vi "Measuring Complete - AndreTec-4.vi"() -> ()   [LabVIEW 2014]
doc: "André Romero - 2016\nandretec@ifsc.usp.br\nIFSC - USP"
uses:
  <vilib>/Analysis/Matrix/Datatypes/RealMatrix.ctl
  C:/UserLabs/Andre/Nova-Autolab/Labview/Autolab SDK 1.11/EcoChemie.Autolab.Sdk.dll
  EcoChemie.Autolab.Sdk.dll
  <vilib>/Instr/_visa.llb/VISA Configure Serial Port (Instr).vi
  <vilib>/Utility/file.llb/Write To Spreadsheet File (DBL).vi
  <vilib>/Analysis/Matrix/NI_Matrix.lvlib
panel:
  in  "String":string="Wait !!!! Instrument is initializing ...."
  in  "Start Measurement":bool
  out "Sensor":i32=1
  out "error out":errorcluster={"status"=TRUE, "code"=-1073807343, "source"="Property Node (arg 1) in VISA Configure Serial Port (Instr).vi->Measuring Complete - AndreTec-2.vi"}
  out "VISA resource name out":refnum<visa-resource-name>="COM3"
  in  "N. Sensors":i32=3 min=1 max=8
  out "Measurement":cluster{dbl[], dbl[]}(graph)
  out "Points":i32=478
  in  "Abort":bool
  in  "Y axis Signal":string(combo)="WE(1).Current"
  in  "X axis Signal":string(combo)="WE(1).Potential"
  out "Measured data":cluster{"Y":dbl[], "Y":dbl[]}[](graph)
  out "X axis value":dbl=-1.1810302734375e-08
  out "Y axis value":dbl=3.0517578124972244e-06
  out "Measurement active":bool
  out "Blacklisted Commands detected":bool
  in  "Load Procedure (.nox)":path=path "C:/Users/user/Documents/My Procedures 1.11/Procedures/bla.nox"
  out "Autolab Connected":bool
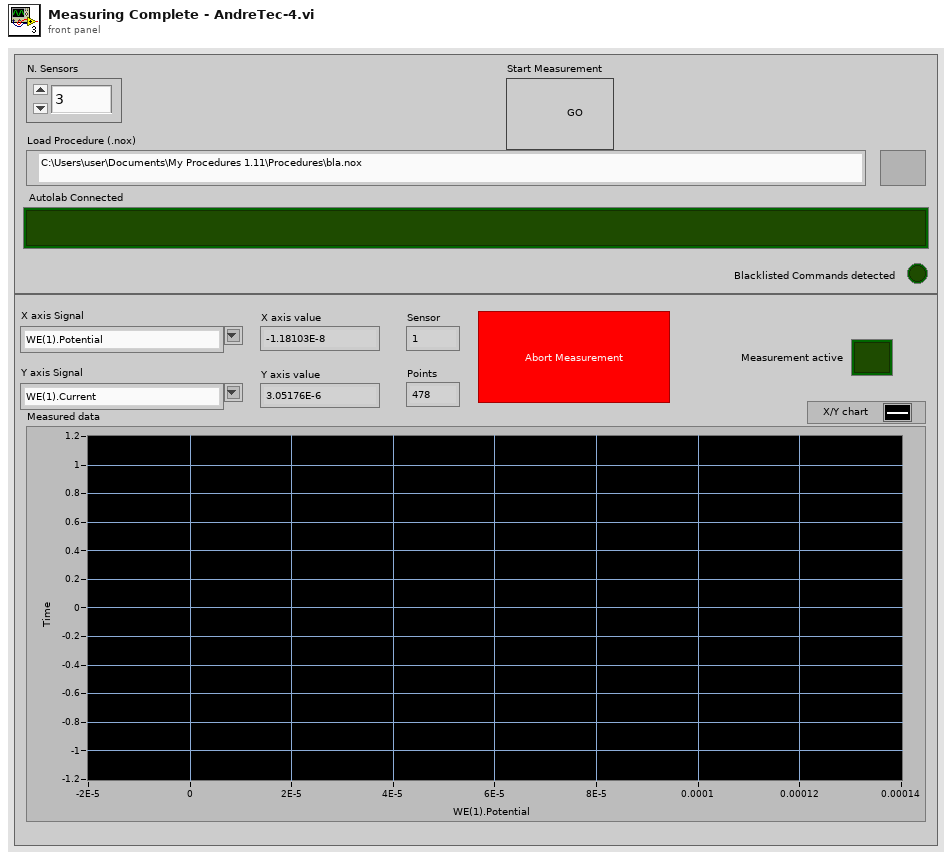
[diagram p1: front panel]
types:
  T1 = typedef "NI_Matrix.lvlib/RealMatrix.ctl" = dbl[][]
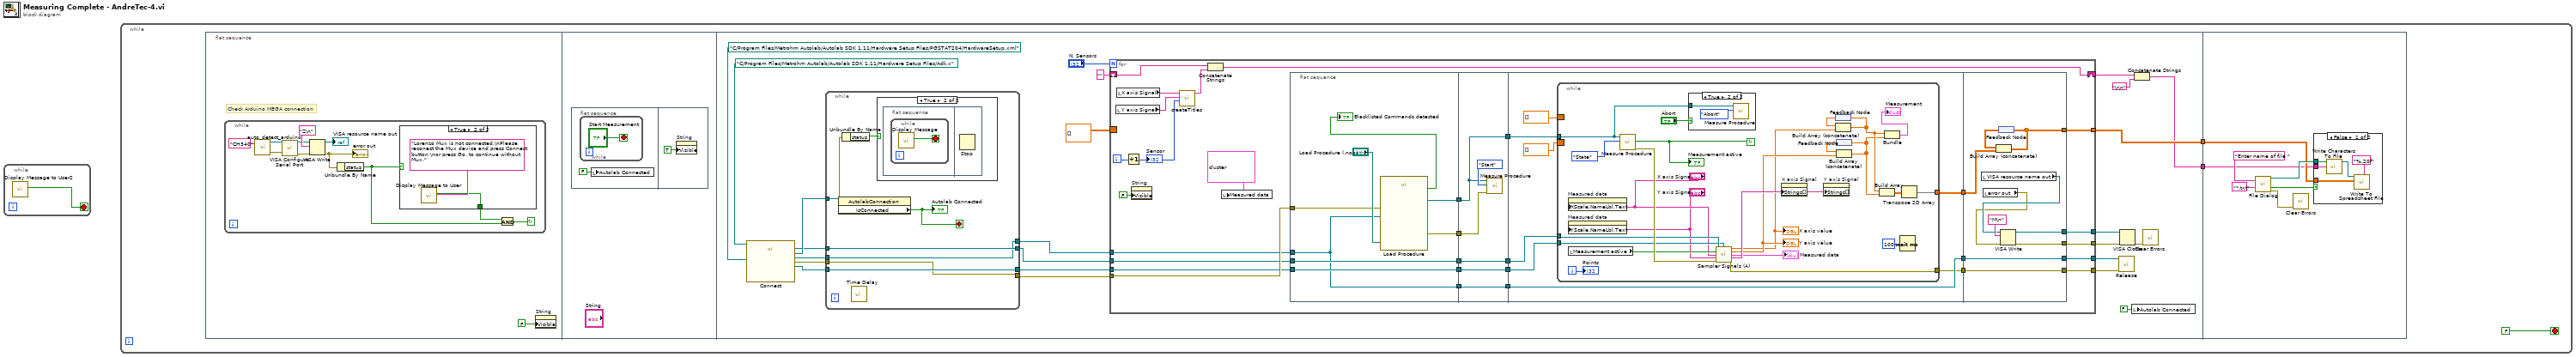
[diagram p0: block diagram]
diagram:
  n1 = while {
    stop <- w1 stop-if-true
    n2 = call "Display Message to User2"() -> ("OK"=w1:bool)  [unwired: 10 in, 1 out]
  }
  n3 = while {
    stop <- FALSE stop-if-true
    n4 = flat-sequence {
      tunnel: [w25] -> w3
      tunnel: [w23] -> w2
      tunnel: w3 -> [w146]
      tunnel: w2 -> [w145]
      frame #0 {
        # "Check Arduino MEGA connection"
        n5 = while {
          stop <- w8 continue-if-true
          n6 = call "auto_detect_arduino.vi"("instr name"="CH340") -> ("VISA resource name"=w16:refnum<visa-resource-name>, "error out"=w9:errorcluster)  [unwired: 1 in, 1 out]
          n7 = call-poly "VISA Configure Serial Port"("VISA resource name"=w16, "error in (no error)"=w9) -> ("VISA resource name out"=w13:refnum<visa-resource-name>, "error out"=w12:errorcluster)  [unwired: 7 in, 5 out]
          n8 = VISA Write(VISA resource name=w13, write buffer="Z\n" ("Command"), error in (no error)=w12) -> (VISA resource name out=→"VISA resource name out":refnum<visa-resource-name>, error out=w10:errorcluster)  [unwired: 1 out]
          "error out" <- w10
          n9 = Unbundle By Name(w10) -> ("status"=w7:bool)
          n10 = case shown="True" w7 {
            tunnel: [_ w17] -> w6
            frame False {
            }
            frame True {
              n11 = call "Display Message to User"("Message"="Lorenzo Mux is not connected.\nPlease reconect the Mux device and press Connect button \nor press Go, to continue without Mux.") -> ("Connect"=w17:bool)  [unwired: 9 in, 1 out]
            }
          }
          n12 = And(x=w6, y=w7) -> (x .and. y?=w8:bool)
        }
        n13 = property on="String" class="Str"("Visible"=FALSE) -> ()  [unwired: 2 in, 2 out]
      }
      frame #1 {
        n14 = flat-sequence {
          frame #0 {
            n15 = while {
              stop <- "Start Measurement" stop-if-true
            }
            n16 = local write "Autolab Connected"(FALSE ("Autolab Connected")) -> ()
          }
          frame #1 {
            n17 = property on="String" class="Str"("Visible"=TRUE) -> ()  [unwired: 2 in, 2 out]
          }
        }
      }
      frame #2 {
        n18 = call "Connect.vi"("Embedded Exe File"=path "C:/Program Files/Metrohm Autolab/Autolab SDK 1.11/Hardware Setup Files/Adk.x", "Hardware Setup File"=path "C:/Program Files/Metrohm Autolab/Autolab SDK 1.11/Hardware Setup Files/PGSTAT204/HardwareSetup.xml") -> ("Sampler"=w42:refnum<k24>, "AutolabConnection"=w43:refnum<k24>, "instrument"=w40:refnum<k24>, "Ei"=w35:refnum<k24>, "error out"=w37:errorcluster)  [unwired: 1 in, 8 out]
        n19 = while {
          tunnel: w43 -> [w140]
          tunnel: w42 -> [w137]
          tunnel: [w137] -> w41
          tunnel: w40 -> [w136]
          tunnel: [w136] -> w39
          tunnel: w35 -> [w135]
          tunnel: [w135] -> w38
          tunnel: w37 -> [w134]
          tunnel: [w134] -> w36
          stop <- w141 stop-if-true
          n20 = property class="AutolabConnection"(reference=w140) -> (error out=w138:errorcluster, "IsConnected"=w141:bool)  [unwired: 1 in, 1 out]
          "Autolab Connected" <- w141
          n21 = Unbundle By Name(w138) -> ("status"=w139:bool)
          n22 = call "Time Delay"() -> ()  [unwired: 2 in, 10 out]
          n23 = case shown="True" w139 {
            frame False {
            }
            frame True {
              n24 = flat-sequence {
                frame #0 {
                  n25 = while {
                    stop <- w142 stop-if-true
                    n26 = call "Display Message"() -> ("OK"=w142:bool)  [unwired: 10 in, 1 out]
                  }
                }
                frame #1 {
                  n27 = Stop() -> ()  [unwired: 1 in]
                }
              }
            }
          }
        }
        n28 = for {
          N: "N. Sensors" -> [_]
          tunnel: [w64] -> w34
          tunnel: [w63] -> w33
          tunnel: [w62] -> w30
          tunnel: [w61] -> w29
          tunnel: w36 -> [w60]
          tunnel: w39 -> [w59]
          tunnel: w41 -> [w58]
          tunnel: w38 -> [w57]
          tunnel: [w54] -> w25
          border: T1 [] ("Real Matrix") -> [_]
          shift-right: [w47] -> w24
          shift-left: "" -> [w49]
          i -> [w53]
          n29 = local read "Y axis Signal"() -> (w50:string)
          n30 = local read "X axis Signal"() -> (w51:string)
          n31 = Increment(x=w53) -> (x+1=w46:i32)
          "Sensor" <- w46
          n32 = property on="String" class="Str"("Visible"=FALSE) -> ()  [unwired: 2 in, 2 out]
          n33 = call "createTitles.vi"("Numeric"=w46, "Y axis Signal"=w50, "X axis Signal"=w51) -> ("String"=w48:string)  [unwired: 8 in]
          n34 = Concatenate Strings(w49, w48) -> (w47:string)
          n35 = local write "Measured data"(cluster{"Y":dbl[], "Y":dbl[]}[] [{"Y"=array[2393 elements], "Y"=array[2393 elements]}] ("Measured data")) -> ()
          n36 = flat-sequence {
            tunnel: [w81] -> w75
            tunnel: [w80] -> w74
            tunnel: [w78] -> w73
            tunnel: [w77] -> w72
            tunnel: [w76] -> w71
            tunnel: w59 -> [w76]
            tunnel: w60 -> [w79]
            tunnel: w58 -> [w78]
            tunnel: w57 -> [w77]
            tunnel: w75 -> [w87]
            tunnel: w74 -> [w88]
            tunnel: [w87] -> w70
            tunnel: w73 -> [w86]
            tunnel: w72 -> [w85]
            tunnel: [w86] -> w69
            tunnel: [w85] -> w68
            tunnel: [w84] -> w67
            tunnel: w71 -> [w84]
            tunnel: w70 -> [w97]
            tunnel: w69 -> [w96]
            tunnel: w68 -> [w95]
            tunnel: w67 -> [w94]
            tunnel: [w94] -> w66
            tunnel: [w90] -> w65
            tunnel: [w93] -> w55
            tunnel: w66 -> [w133]
            tunnel: w65 -> [w132]
            tunnel: [w133] -> w64
            tunnel: [w132] -> w63
            tunnel: [w128] -> w62
            tunnel: [w127] -> w61
            tunnel: w55 -> [w126]
            tunnel: [w124] -> w54
            frame #0 {
              n37 = call "Load Procedure.vi"("error in (no error)"=w79, "Procedure"="Load Procedure (.nox)", "Instrument"=w76) -> ("error out"=w80:errorcluster, "Contains"=→"Blacklisted Commands detected":bool, "LoadProcedure"=w81:refnum<k24>)  [unwired: 6 out]
            }
            frame #1 {
              n38 = call "Measure Procedure.vi"("error in"=w88, "Request for procedure"=enum16{"State", "Save", "Abort", "Start"}."Start", "LoadProcedure"=w87) -> ()  [unwired: 1 in, 8 out]
            }
            frame #2 {
              n39 = while {
                tunnel: w97 -> [w115]
                tunnel: w96 -> [w116]
                tunnel: w95 -> [w100]
                tunnel: [w103] -> w93
                border: dbl[] [] -> [_]
                border: dbl[] [] -> [_]
                tunnel: [w102] -> w90
                i -> [w112]
                stop <- w107 continue-if-true
                n40 = property on="Measured data" class="XYGraph (strict)"("XScale.NameLbl.Text"="X axis Signal") -> ()  [unwired: 2 in, 2 out]
                n41 = property on="Measured data" class="XYGraph (strict)"("YScale.NameLbl.Text"="Y axis Signal") -> ()  [unwired: 2 in, 2 out]
                n42 = local read "Measurement active"() -> (w118:bool)
                n43 = call "Measure Procedure.vi"("Request for procedure"=enum16{"State", "Save", "Abort", "Start"}."State", "LoadProcedure"=w115) -> ("error out"=w119:errorcluster, "IsMeasuring"=w107:bool)  [unwired: 2 in, 6 out]
                "Measurement active" <- w107
                n44 = case shown="True" "Abort" {
                  tunnel: w115 -> [_ w122]
                  frame False {
                  }
                  frame True {
                    n45 = call "Measure Procedure.vi"("Request for procedure"=enum16{"State", "Save", "Abort", "Start"}."Abort", "LoadProcedure"=w122) -> ()  [unwired: 2 in, 8 out]
                  }
                }
                n46 = call "Sampler Signals (A).vi"("IsMeasuring"=w118, "EI"=w100, "Sampler"=w116, "Signal X"="X axis Signal", "Signal Y"="Y axis Signal", "error in"=w119) -> ("X"=w101:dbl, "Y"=w109:dbl, "XY Graph"=→"Measured data":cluster{"Y":dbl[], "Y":dbl[]}[], "GetSignals"=w121:string[], "error out"=w102:errorcluster)  [unwired: 4 in, 1 out]
                "Y axis value" <- w109
                "X axis value" <- w101
                n47 = property on="X axis Signal" class="CmbBox"("Strings[]"=w121) -> ()  [unwired: 2 in, 2 out]
                n48 = property on="Y axis Signal" class="CmbBox"("Strings[]"=w121) -> ()  [unwired: 2 in, 2 out]
                n49 = feedback #1() -> (w111:dbl[])
                n50 = Build Array (concatenate)(w111, w101) -> (w105:dbl[])
                n51 = feedback-in #1(w105) -> ()
                n52 = feedback #2() -> (w110:dbl[])
                n53 = Build Array (concatenate)(w110, w109) -> (w104:dbl[])
                n54 = feedback-in #2(w104) -> ()
                n55 = Build Array(w105, w104) -> (w106:dbl[][])
                n56 = Bundle(w105, w104) -> (→"Measurement":cluster{dbl[], dbl[]})  [unwired: 1 in]
                n57 = Wait (ms)(milliseconds to wait=u32 100) -> ()  [unwired: 1 out]
                n58 = Transpose 2D Array(2D array=w106) -> (transposed array=w103:dbl[][])
                "Points" <- w112
              }
            }
            frame #3 {
              n59 = local read "VISA resource name out"() -> (w130:refnum<visa-resource-name>)
              n60 = local read "error out"() -> (w129:errorcluster)
              n61 = feedback #3() -> (w125:T1)
              n62 = Build Array (concatenate)(w125, w126) -> (w124:T1)
              n63 = feedback-in #3(w124) -> ()
              n64 = VISA Write(VISA resource name=w130, write buffer="M\n" ("Command"), error in (no error)=w129) -> (VISA resource name out=w128:refnum<visa-resource-name>, error out=w127:errorcluster)  [unwired: 1 out]
            }
          }
        }
        n65 = call "Release.vi"("error in (no error)"=w33, "Instrument"=w34) -> ()  [unwired: 1 in, 9 out]
        n66 = VISA Close(VISA resource name=w30, error in (no error)=w29) -> (error out=w31:errorcluster)
        n67 = local write "Autolab Connected"(FALSE ("Autolab Connected")) -> ()
        n68 = Concatenate Strings(w24, "\r\n") -> (w23:string)
        n69 = call <vilib>:"Clear Errors.vi"("error in (no error)"=w31) -> ()  [unwired: 5 in, 2 out]
      }
      frame #3 {
        n70 = call "File Dialog"("prompt"="Enter name of file ", "pattern (all files)"="*.txt") -> ("selected path"=w147:path, "cancelled"=w143:bool, "error out"=w144:errorcluster)  [unwired: 10 in, 1 out]
        n71 = call <vilib>:"Clear Errors.vi"("error in (no error)"=w144) -> ()  [unwired: 5 in, 2 out]
        n72 = case shown="False" w143 {
          tunnel: w147 -> [w154 _]
          tunnel: w146 -> [w151 _]
          tunnel: w145 -> [w150 _]
          frame False {
            n73 = call <vilib>:"Write Characters To File.vi"("character string"=w150, "file path (dialog if empty)"=w154) -> ("new file path (Not A Path if cancelled)"=w153:path)  [unwired: 3 in]
            n74 = call-poly <vilib>:"Write To Spreadsheet File.vi"("format (%.3f)"="%.20f", "2D data"=w151, "file path (dialog if empty)"=w153) -> ()  [unwired: 5 in, 1 out]
          }
          frame True {
          }
        }
      }
    }
  }
